vi "Derive Target Method Name.vi"(8 "error in (no error)":errorcluster, 11 "Library":refnum<vi>) -> (0 "error out":errorcluster, 2 "Likely Target Method":string)   [LabVIEW 2020, in "Message Rescripter.lvlib"]
uses:
  Message Rescripter.lvlib
  <vilib>/Utility/traverseref.llb/VI Scripting - Traverse.lvlib
  <vilib>/Utility/traverseref.llb/TRef TravTarget.ctl
  <vilib>/ErrorRing/Error Ring.xnode
  <vilib>/Utility/error.llb/Error Cluster From Error Code.vi
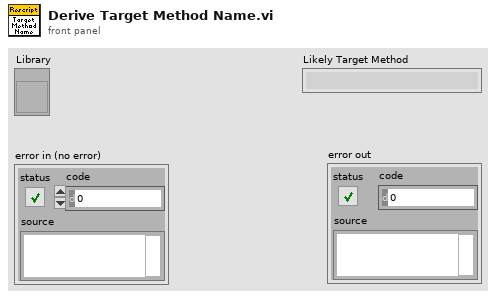
[diagram p1: front panel]
types:
  T1 = typedef "TRef TravTarget.ctl" = enum16{"FP", "BD", "Other"}
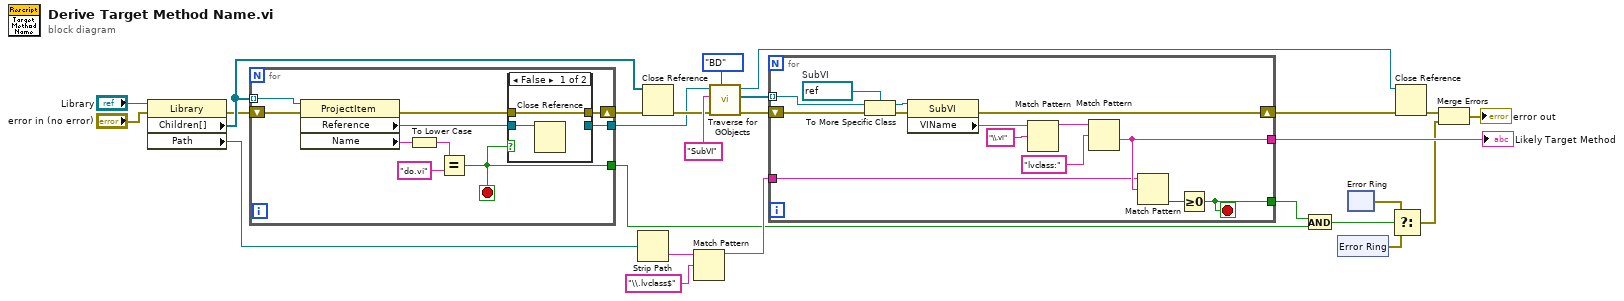
[diagram p0: block diagram]
diagram:
  n1 = property class="Library"(reference="Library", error in="error in (no error)") -> (error out=w9:errorcluster, "Children[]"=w25:refnum<vi>[], "Path"=w8:path)  [unwired: 1 out]
  n2 = for {
    tunnel: w25 -> [w36] mode=indexing
    shift-right: [w27] -> w24
    shift-left: w9 -> [w35]
    tunnel: [w29] -> w6
    tunnel: [w31] -> w14
    stop <- w31 stop-if-true
    n3 = property class="ProjectItem"(reference=w36, error in=w35) -> (error out=w28:errorcluster, "Reference"=w30:refnum<vi>, "Name"=w34:string)  [unwired: 1 out]
    n4 = To Lower Case(string=w34) -> (all lower case string=w32:string)
    n5 = Equal?(x=w32, y="do.vi" ("element")) -> (x = y?=w31:bool)
    n6 = case shown="False" w31 {
      tunnel: [_ w40] -> w29
      tunnel: w30 -> [w38 w40]
      tunnel: [w37 w39] -> w27
      tunnel: w28 -> [w37 w39]
      frame False {
        n7 = Close Reference(reference=w38) -> ()  [unwired: 1 in, 1 out]
      }
      frame True {
      }
    }
  }
  n8 = Strip Path(path=w8) -> (name=w19:string)  [unwired: 1 out]
  n9 = Close Reference(reference=w25, error in (no error)=w24) -> (error out=w21:errorcluster)
  n10 = Match Pattern(string=w19, regular expression="\\.lvclass$") -> (before substring=w17:string)  [unwired: 1 in, 3 out]
  n11 = call <vilib>:"Traverse for GObjects.vi"("Traverse Target"=TRef_TravTarget."BD", "error in (no error)"=w21, "Class Name"="SubVI", "VI Refnum"=w6) -> ("error out"=w5:errorcluster, "References"=w4:refnum<vi>[], "dup VI Refnum"=w1:refnum<vi>)  [unwired: 4 in, 1 out]
  n12 = for {
    tunnel: w4 -> [w54] mode=indexing
    shift-right: [w53] -> w20
    shift-left: w5 -> [w51]
    tunnel: [w44] -> w16
    tunnel: w17 -> [w41]
    tunnel: [w42] -> w15
    stop <- w42 stop-if-true
    w49 = refnum<vi> refnum  # SubVI
    n13 = To More Specific Class(target class=w49, reference=w54, error in=w51) -> (specific class reference=w52:refnum<vi>, error out=w50:errorcluster)
    n14 = property class="SubVI"(reference=w52, error in=w50) -> (error out=w53:errorcluster, "VIName"=w45:string)  [unwired: 1 out]
    n15 = Match Pattern(string=w45, regular expression="\\.vi") -> (before substring=w48:string)  [unwired: 1 in, 3 out]
    n16 = Match Pattern(string=w48, regular expression="lvclass:") -> (after substring=w44:string)  [unwired: 1 in, 3 out]
    n17 = Match Pattern(string=w41, regular expression=w44) -> (offset past match=w43:i32)  [unwired: 1 in, 3 out]
    n18 = Greater Or Equal To 0?(x=w43) -> (x >= 0?=w42:bool)
  }
  "Likely Target Method" <- w16
  n19 = And(x=w15, y=w14) -> (x .and. y?=w13:bool)
  n20 = xnode "Error Ring"() -> ("error out"=w3:errorcluster)
  n21 = xnode "Error Ring"() -> ("error out"=w2:errorcluster)
  n22 = Select(t=w2, s=w13, f=w3) -> (s? t:f=w10:errorcluster)
  n23 = Close Reference(reference=w1, error in (no error)=w20) -> (error out=w12:errorcluster)
  n24 = Merge Errors(w12, w10) -> (→"error out":errorcluster)
